vi "Sensor Port Mapping Global.vi"(8 "Action":T3, 9 "Ports":u32[](array[numeric]), 10 "Thermocouple?":bool[](array[boolean]), 11 "Sensors":T2[](array[typedef])) -> (2 "Mapping List":T1[](array[typedef]))   [LabVIEW 2015]
uses:
  Sensor Port Mapping Global Action.ctl
  Sensor Enum.ctl
  Sensor Port Mapping.ctl
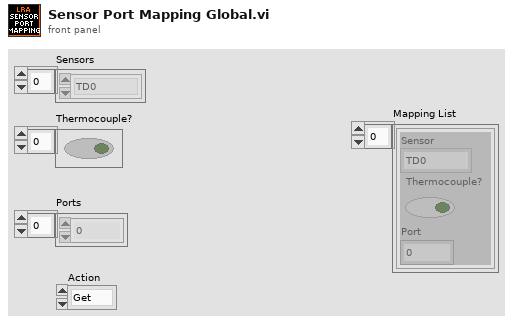
[diagram p1: front panel]
types:
  T1 = typedef "Sensor Port Mapping.ctl" = cluster{"Sensor":T2, "Thermocouple?":bool, "Port":u32}
  T2 = typedef "Sensor Enum.ctl" = enum16{"TD0", "TD1", "TD2", "TD3", "TD4", "TD5", "TD6", "TD7", "TD8", "TD9", "TD10"}
  T3 = typedef "Sensor Port Mapping Global Action.ctl" = enum16{"Get", "Set"}
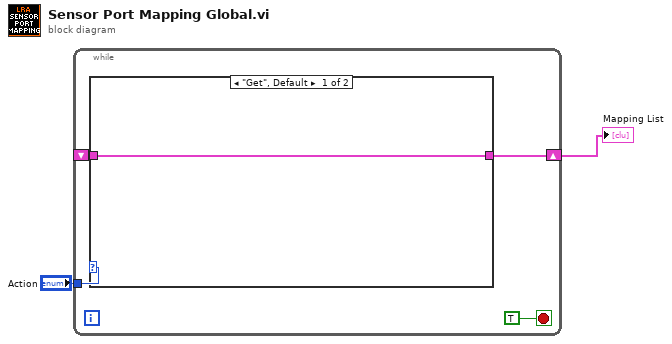
[diagram p0: block diagram]
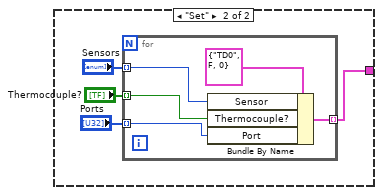
[diagram p2: hidden frame]
diagram:
  n1 = while {
    tunnel: "Action" -> [w5]
    shift-right: [w3] -> w1
    shift-left: _ -> [w4]
    stop <- TRUE stop-if-true
    n2 = case shown="\"Get\", Default" w5 {
      tunnel: w4 -> [w7 _]
      tunnel: [w7 w8] -> w3
      frame "Get", Default {
      }
      frame "Set" {
        n3 = for {
          tunnel: "Ports" -> [w15] mode=indexing
          tunnel: "Thermocouple?" -> [w14] mode=indexing
          tunnel: "Sensors" -> [w13] mode=indexing
          tunnel: [w12] -> w8 mode=indexing
          n4 = Bundle By Name(cluster=T1 {"Sensor"=enum."TD0", "Thermocouple?"=FALSE, "Port"=0} ("Cluster"), "Sensor"=w13, "Thermocouple?"=w14, "Port"=w15) -> (w12:T1)
        }
      }
    }
  }
  "Mapping List" <- w1
